vi "copyScriptToRunDirLoop.vi"(8 "error in (no error)":errorcluster, 10 "Path in":path, 11 "FileNeologist in":refnum<class "FileNeologist.lvclass">) -> (0 "error out":errorcluster, 2 "Path out":path, 3 "FileNeologist out":refnum<class "FileNeologist.lvclass">)   [LabVIEW 2009, in "Tools.lvlib" / "Filing.lvlib" / "FileNeologist.lvclass"]
uses:
  FileNeologist.lvclass
  FileNeologist.lvclass/FileNeologist.ctl
panel:
  out "out":string
  out "in":string
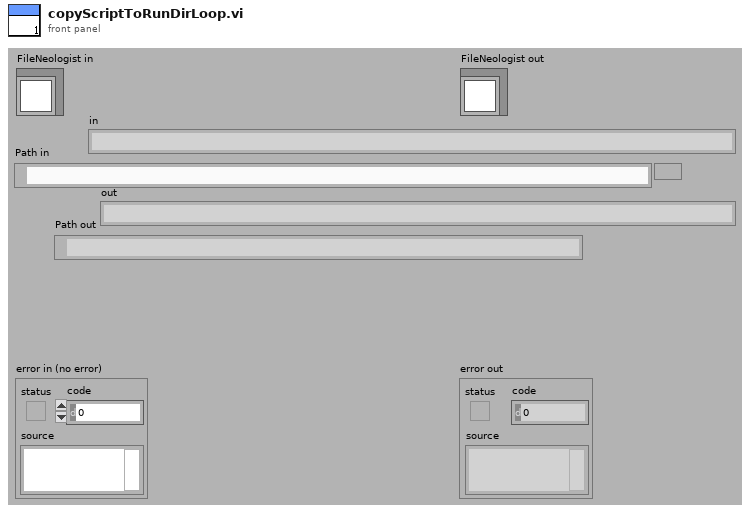
[diagram p1: front panel]
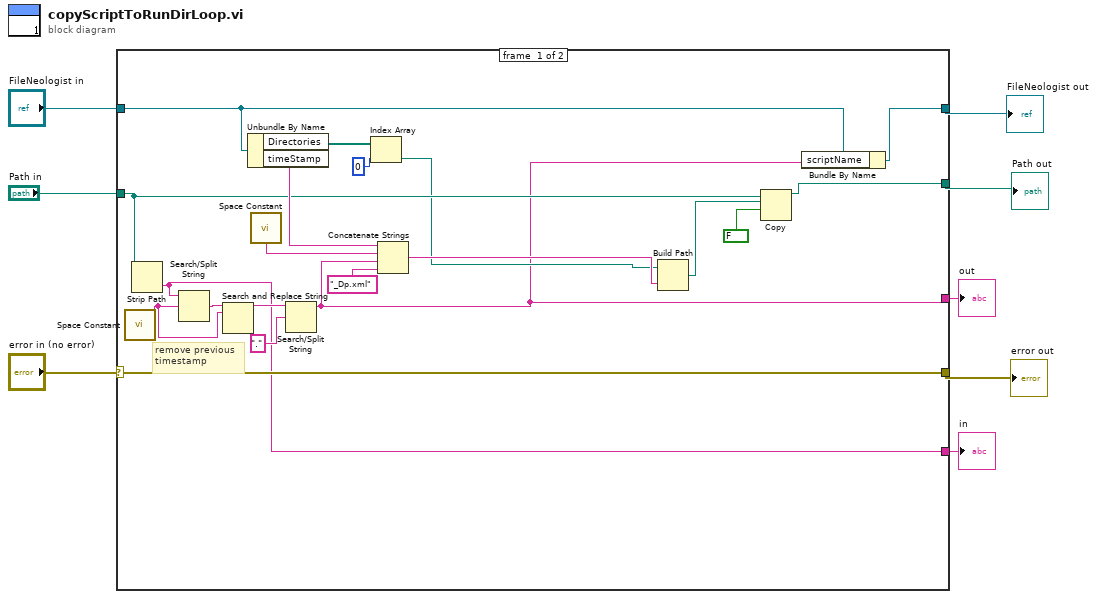
[diagram p0: block diagram]
diagram:
  n1 = case shown="No Error" "error in (no error)" {
    selector: "error in (no error)" -> [w15 w30]
    tunnel: [w15 w30] -> w7
    tunnel: [w18 w29] -> w5
    tunnel: "FileNeologist in" -> [w19 w29]
    tunnel: "Path in" -> [w23 _]
    tunnel: [w22 _] -> w3
    tunnel: [w10 _] -> w2
    tunnel: [w9 _] -> w1
    frame #0 {
      # "remove previous\ntimestamp"
      n2 = call <vilib>:"Space Constant.vi"() -> ("String"=w12:string)
      n3 = Strip Path(path=w23) -> (name=w10:string)  [unwired: 1 out]
      n4 = Search/Split String(string=w10, search string/char (-)=w12) -> (match + rest of string=w13:string)  [unwired: 1 in, 2 out]
      n5 = Search and Replace String(input string=w13, search string=w12) -> (result string=w11:string)  [unwired: 6 in, 3 out]
      n6 = Unbundle By Name(w19) -> ("Directories"=w21:path[], "timeStamp"=w24:string)
      n7 = call <vilib>:"Space Constant.vi"() -> ("String"=w26:string)
      n8 = Search/Split String(string=w11, search string/char (-)=".") -> (substring before match=w9:string)  [unwired: 1 in, 2 out]
      n9 = Index Array(array=w21, index=0) -> (element=w16:path)
      n10 = Concatenate Strings(w24, w26, w9, "_Dp.xml") -> (w20:string)
      n11 = Build Path(base path=w16, name or relative path=w20) -> (appended path=w25:path)
      n12 = Copy(9:FALSE, 10:w25, 11:w23) -> (3:w22:path)  [unwired: 2 in, 2 out]
      n13 = Bundle By Name(cluster=w19, "scriptName"=w9) -> (w18:refnum<class "FileNeologist.lvclass">)
    }
    frame #1 {
    }
  }
  "error out" <- w7
  "FileNeologist out" <- w5
  "Path out" <- w3
  "in" <- w2
  "out" <- w1
